vi "Read Waveform From File.vi"(0 "VISA resource name":refnum<visa-resource-name>, 1 "Skip N Points (1)":i32=1, 5 "Start Point (1)":i32=1, 7 "End Point (10000)":i32=10000, 9 "Filename (C:\\data.txt)":path=path "C:/data.txt", 11 "error in (no error)":errorcluster) -> (4 "VISA resource name out":refnum<visa-resource-name>, 6 "Waveform Graph":waveform(sgl)(graph), 8 "Time Interval":sgl, 10 "Count":i32, 14 "Start Time":sgl, 15 "error out":errorcluster)   [LabVIEW 2015, in "Tektronix 7000 Series.lvlib"]
doc: "Reads the sample points between the starting and ending positions of waveform data in a file that you specify. The computer will have limitations on the amount of data that can be read. You can skip some points in order to read successfully."
uses:
  <instrlib>/Tektronix 7000 Series/Tektronix 7000 Series.lvlib
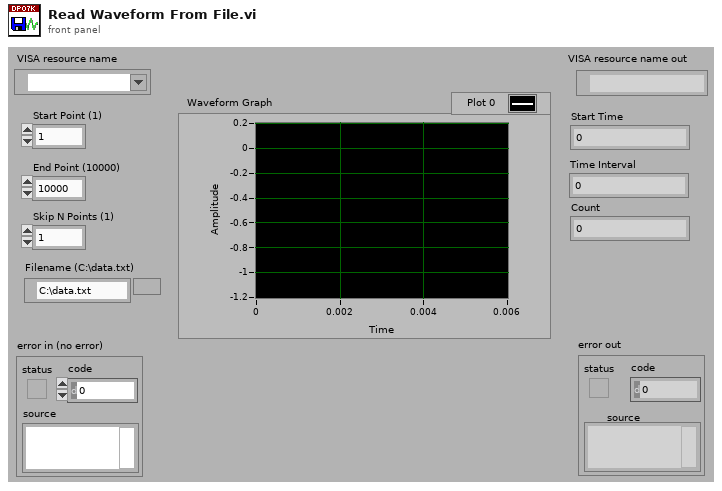
[diagram p1: front panel]
types:
  T1 = enum16{"open", "open or create", "create or replace", "create", "open (read only)"}
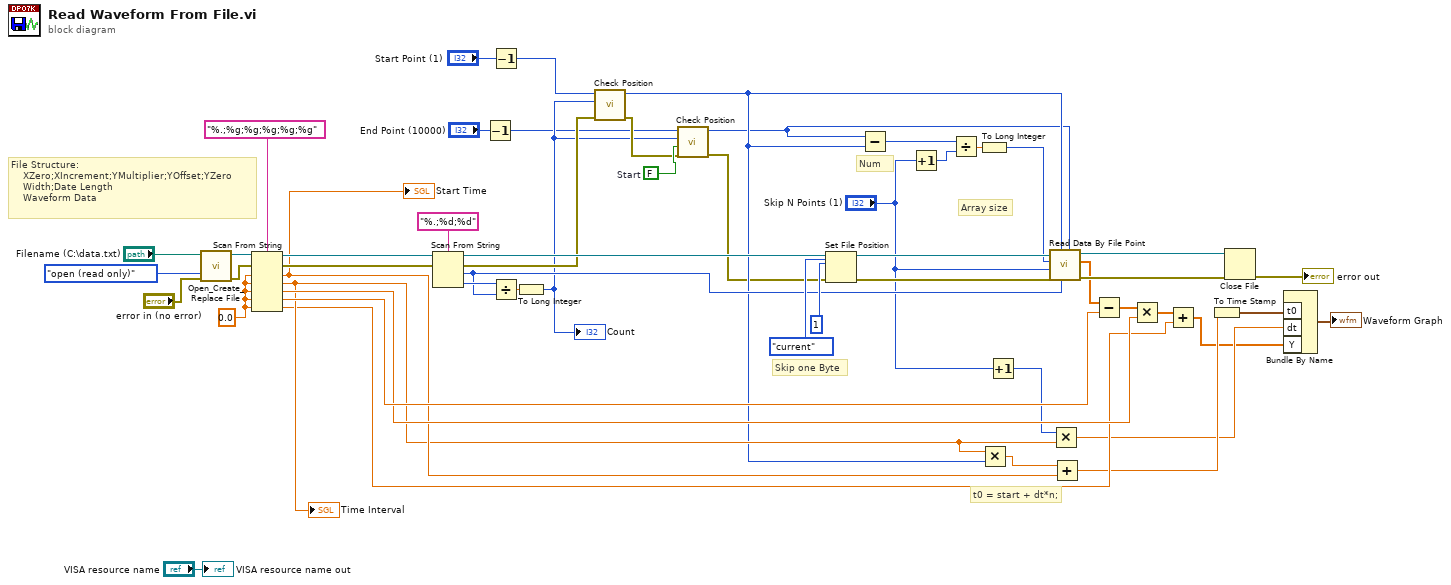
[diagram p0: block diagram]
diagram:
  w12 = FALSE  # Start
  w25 = sgl 0.0 ("t")
  # "Array size"
  # "Num"
  # "File Structure:\n    XZero;XIncrement;YMultiplier;YOffset;YZero\n    Width;Date Length\n    Waveform Data"
  # "t0 = start + dt*n;"
  # "Skip one Byte"
  n1 = call <vilib>:"Open_Create_Replace File.vi"("error in (no error)"="error in (no error)", "function (open:0)"=T1."open (read only)", "file path"="Filename (C:\\data.txt)") -> ("error out"=w30:errorcluster, "refnum"=w51:refnum<file>)  [unwired: 5 in, 2 out]
  n2 = Scan From String ("Scan From File")("%.;%g;%g;%g;%g;%g" ("format string"), w51, w30, default 1=w25, default 2=w25, default 3=w25, default 4=w25, default 5=w25) -> (w49:refnum<file>, w48:errorcluster, output 1=w41:sgl, output 2=w26:sgl, output 3=w44:sgl, output 4=w45:sgl, output 5=w23:sgl)
  "Start Time" <- w41
  "Time Interval" <- w26
  n3 = Scan From String ("Scan From File")("%.;%d;%d" ("format string"), w49, w48) -> (w40:refnum<file>, w13:errorcluster, output 1=w27:i32, output 2=w31:i32)  [unwired: 2 in]
  n4 = Decrement(x="End Point (10000)") -> (x-1=w9:i32)
  n5 = Decrement(x="Start Point (1)") -> (x-1=w14:i32)
  n6 = Divide(x=w31, y=w27) -> (x/y=w28:dbl)
  n7 = To Long Integer(number=w28) -> (32bit integer=w10:i32)
  "Count" <- w10
  n8 = call <instrlib>:"Check Position.vi"("error in (no error)"=w13, "Count (10000)"=w10, "Point In (0)"=w14) -> ("error out"=w11:errorcluster, "Point Out"=w8:i32)  [unwired: 7 in]
  n9 = call <instrlib>:"Check Position.vi"("error in (no error)"=w11, "Start (True)"=w12, "Count (10000)"=w10, "Point In (0)"=w9) -> ("error out"=w7:errorcluster, "Point Out"=w6:i32)  [unwired: 6 in]
  n10 = Set File Position(offset (in bytes) (0)=1 ("pos offset (0)"), refnum=w40, from (0:start)=enum16{"start", "end", "current"}."current" ("pos mode (0:2)"), error in=w7) -> (refnum out=w37:refnum<file>, error out=w36:errorcluster)
  n11 = Subtract(x=w6, y=w8) -> (x-y=w17:i32)
  n12 = Increment(x="Skip N Points (1)") -> (x+1=w16:i32)
  n13 = Divide(x=w17, y=w16) -> (x/y=w18:dbl)
  n14 = To Long Integer(number=w18) -> (32bit integer=w15:i32)
  n15 = Multiply(x=w26, y=w8) -> (x*y=w33:sgl)
  n16 = Increment(x="Skip N Points (1)") -> (x+1=w22:i32)
  n17 = call <instrlib>:"Read Data By File Point.vi"("End Point"=w6, "Data Width"=w27, "Start Point"=w8, "error in"=w36, "Skip N Points"="Skip N Points (1)", "Dimension Size"=w15, "Byte Stream File Refnum In"=w37) -> ("error out"=w34:errorcluster, "Array"=w32:sgl[], "Byte Stream File Refnum Out"=w35:refnum<file>)  [unwired: 2 in]
  n18 = Multiply(x=w22, y=w26) -> (x*y=w3:sgl)
  n19 = Add(x=w33, y=w41) -> (x+y=w4:sgl)
  n20 = Subtract(x=w32, y=w45) -> (x-y=w42:sgl[])
  n21 = Multiply(x=w42, y=w44) -> (x*y=w24:sgl[])
  n22 = Add(x=w24, y=w23) -> (x+y=w2:sgl[])
  n23 = To Time Stamp(1:w4) -> (0:w5:timestamp)
  n24 = Close File(refnum=w35, error in=w34) -> (error out=→"error out":errorcluster)  [unwired: 1 out]
  n25 = Bundle By Name ("Build Waveform")("t0"=w5, "dt"=w3, "Y"=w2) -> (→"Waveform Graph":waveform(sgl))  [unwired: 1 in]
  "VISA resource name out" <- "VISA resource name"
